vi "dfd_Halfband Filter Design.vi"(5 "method":u16(ring) items=["Kaiser Window", "Dolph-Chebyshev Window", "Equi-Ripple", "Positive Equi-Ripple"], 7 "filter type":enum16{"Lowpass", "Highpass"}(ring), 8 "error IO":errorcluster, 10 "roll off":dbl, 11 "order":i32) -> (0 "error out":errorcluster, 2 "order out":i32, 3 "h out":dbl[](array[numeric]))   [LabVIEW 2017, in "NI_DigFilter_Process.lvlib"]
uses:
  <vilib>/addons/Digital Filter Design/NI_DigFilter_Process.lvlib
  <vilib>/addons/Digital Filter Design/_REMEZ.llb/remez_fir filter type.ctl
  <vilib>/addons/Digital Filter Design/NI_DigFilter_Design.lvlib
  <vilib>/addons/Digital Filter Design/NI_DigFilterLicensed.lvlib
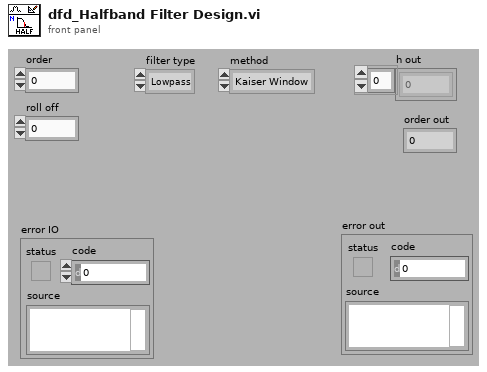
[diagram p1: front panel]
types:
  T1 = typedef "NI_DigFilterLicensed.lvlib/remez_fir filter type.ctl" = enum32{"Symmetric", "Antisymmetric", "Differentiator", "Hilbert", "Minimum Phase", "Maximum Phase"}
  T2 = typedef "NI_DigFilterLicensed.lvlib/DFD Adv Band Spec.ctl" = cluster{"band specification":cluster{"freq":dbl, "amplitude":dbl, "weight":dbl}[], "ripple constraint":dbl}
  T3 = typedef "remez_band specification.ctl" = T4[]
  T4 = typedef "remez_single band description.ctl" = cluster{"points":cluster{"f":dbl, "A":dbl, "W":dbl, "forced gain?":bool}[], "band weight":dbl, "constraint":dbl, "ripple idx":i32, "in band weight option":enum16{"ignore", "linear interpolation", "const amplitude %"}}
  T5 = typedef "remez_fir order and types.ctl" = cluster{"# of taps":i32, "filter type":T1, "minimum order":enum32{"user defined", "minEven", "minOdd"}}
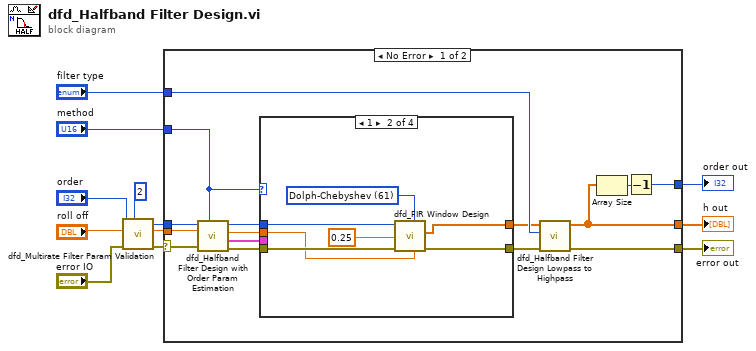
[diagram p0: block diagram]
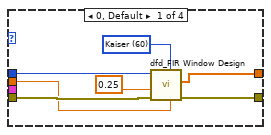
[diagram p2: hidden frame]
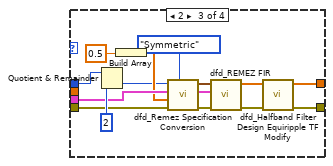
[diagram p3: hidden frame]
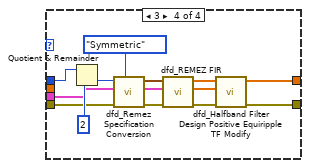
[diagram p4: hidden frame]
diagram:
  n1 = call <vilib>:"dfd_Multirate Filter Param Validation.vi"("multirate factor"=2, "error in (no error)"="error IO", "roll off"="roll off", "order"="order") -> ("error out"=w1:errorcluster, "dup roll off"=w3:dbl, "dup order"=w2:i32)  [unwired: 2 in, 3 out]
  n2 = case shown="No Error" w1 {
    selector: w1 -> [w13 w71]
    tunnel: "method" -> [w27 _]
    tunnel: [w22 w71] -> w11
    tunnel: "filter type" -> [w21 _]
    tunnel: [w17 _] -> w9
    tunnel: [w16 _] -> w8
    tunnel: w3 -> [w15 _]
    tunnel: w2 -> [w14 _]
    frame No Error {
      n3 = call <vilib>:"dfd_Halfband Filter Design with Order Param Estimation.vi"("method"=w27, "error in (no error)"=w13, "roll off"=w15, "order"=w14) -> ("error out"=w25:errorcluster, "band parameters"=w24:T2[], "window param"=w23:dbl, "order out"=w26:i32)  [unwired: 4 out]
      n4 = case shown="1" w27 {
        tunnel: w26 -> [w34 w40 w56 w70]
        tunnel: w23 -> [w31 w36 _ _]
        tunnel: w25 -> [w32 w41 w48 w61]
        tunnel: [w30 w37 w50 w64] -> w19
        tunnel: [w29 w38 w51 w65] -> w20
        tunnel: w24 -> [_ _ w49 w62]
        frame 0, Default {
          w28 = u16 60 items=["None"=0, "Hanning"=1, "Hamming"=2, "Blackman-Harris"=3, "Exact Blackman"=4, "Blackman"=5, "Flat Top"=6, "4 Term B-Harris"=7, "7 Term B-Harris"=8, "Low Sidelobe"=9, "Triangular"=30, "Kaiser"=60, "Dolph-Chebyshev"=61] ("window")
          n5 = call <vilib>:"dfd_FIR Window Design.vi"("param"=w31, "window"=w28, "error in (no error)"=w32, "low cutoff freq: fl"=0.25 ("element"), "order"=w34) -> ("error out"=w30:errorcluster, "h"=w29:dbl[])  [unwired: 3 in, 2 out]
        }
        frame 1 {
          w35 = u16 61 items=["None"=0, "Hanning"=1, "Hamming"=2, "Blackman-Harris"=3, "Exact Blackman"=4, "Blackman"=5, "Flat Top"=6, "4 Term B-Harris"=7, "7 Term B-Harris"=8, "Low Sidelobe"=9, "Triangular"=30, "Kaiser"=60, "Dolph-Chebyshev"=61] ("window")
          n6 = call <vilib>:"dfd_FIR Window Design.vi"("param"=w36, "window"=w35, "error in (no error)"=w41, "low cutoff freq: fl"=0.25 ("element"), "order"=w40) -> ("error out"=w37:errorcluster, "h"=w38:dbl[])  [unwired: 3 in, 2 out]
        }
        frame 2 {
          n7 = Quotient & Remainder(x=w56, y=2) -> (floor(x/y)=w42:i32)  [unwired: 1 out]
          n8 = Build Array(0.5 ("Numeric")) -> (w46:dbl[])
          n9 = call <vilib>:"dfd_Remez Specification Conversion.vi"("phase option"=remez_fir_filter_type."Symmetric" ("filter type"), "error in (no error)"=w48, "freq of forced gain [Hz]"=w46, "band parameters"=w49, "order"=w42) -> ("error out"=w45:errorcluster, "band specification"=w44:T3, "order and type"=w43:T5)  [unwired: 1 in, 3 out]
          n10 = call <vilib>:"dfd_REMEZ FIR.vi"("error in (no error)"=w45, "band specification"=w44, "order and type"=w43) -> ("error out"=w53:errorcluster, "h"=w52:dbl[])  [unwired: 3 in, 4 out]
          n11 = call <vilib>:"dfd_Halfband Filter Design Equiripple TF Modify.vi"("error in (no error)"=w53, "h in"=w52) -> ("error out"=w50:errorcluster, "h out"=w51:dbl[])  [unwired: 1 in, 7 out]
        }
        frame 3 {
          n12 = Quotient & Remainder(x=w70, y=2) -> (floor(x/y)=w63:i32)  [unwired: 1 out]
          n13 = call <vilib>:"dfd_Remez Specification Conversion.vi"("phase option"=remez_fir_filter_type."Symmetric" ("filter type"), "error in (no error)"=w61, "band parameters"=w62, "order"=w63) -> ("error out"=w59:errorcluster, "band specification"=w57:T3, "order and type"=w58:T5)  [unwired: 2 in, 3 out]
          n14 = call <vilib>:"dfd_REMEZ FIR.vi"("error in (no error)"=w59, "band specification"=w57, "order and type"=w58) -> ("error out"=w67:errorcluster, "actual ripples"=w66:dbl[], "h"=w68:dbl[])  [unwired: 2 in, 4 out]
          n15 = call <vilib>:"dfd_Halfband Filter Design Positive Equiripple TF Modify.vi"("error in (no error)"=w67, "actual ripples"=w66, "h in"=w68) -> ("error out"=w64:errorcluster, "h out"=w65:dbl[])  [unwired: 3 in, 4 out]
        }
      }
      n16 = call <vilib>:"dfd_Halfband Filter Design Lowpass to Highpass.vi"("error in (no error)"=w19, "filter type"=w21, "h in"=w20) -> ("error out"=w22:errorcluster, "h out"=w17:dbl[])  [unwired: 7 out]
      n17 = Array Size(array=w17) -> (size(s)=w18:i32)
      n18 = Decrement(x=w18) -> (x-1=w16:i32)
    }
    frame Error {
    }
  }
  "error out" <- w11
  "h out" <- w9
  "order out" <- w8
